vi "ScanAction.vi"(8 "error in (no error)":errorcluster caption="entrée d'erreur (pas d'erreur)", 9 "IndicePoint":i32, 10 "Dir":bool, 11 "Tools In":refnum<class "HeFlowMeter.lvclass"> caption="DNL_LabVIEW Object in") -> (0 "error out":errorcluster caption="sortie d'erreur", 2 "ScanParsOut":dbl[](array[numeric]), 3 "Tools Out":refnum<class "HeFlowMeter.lvclass"> caption="DNL_LabVIEW Object out")   [LabVIEW 2019, in "HeFlowMeter.lvclass"]
uses:
  HeFlowMeter.lvclass
  HeFlowMeter.lvclass/HeFlowMeter.ctl
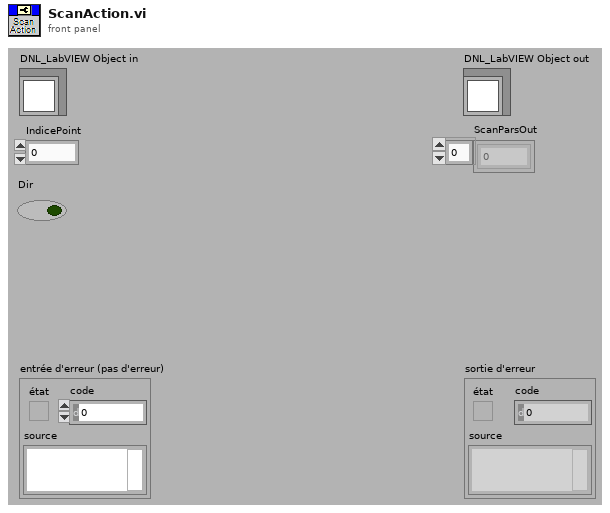
[diagram p1: front panel]
types:
  T1 = typedef "HeFlowMeter.lvclass/HeFlowMeter_Func.ctl" = enum16{"ReadFlow (m3h-1)"}
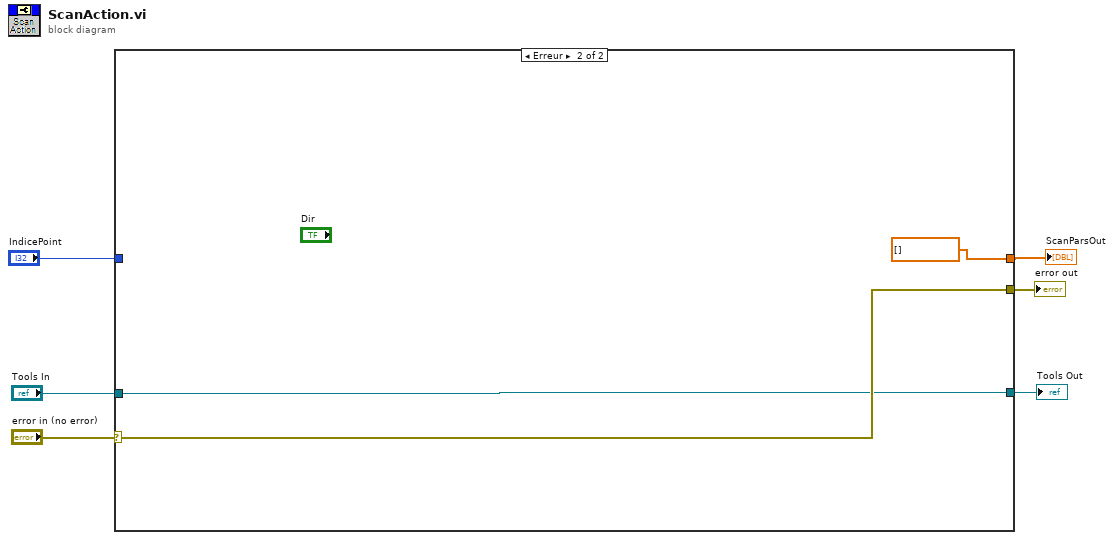
[diagram p0: block diagram]
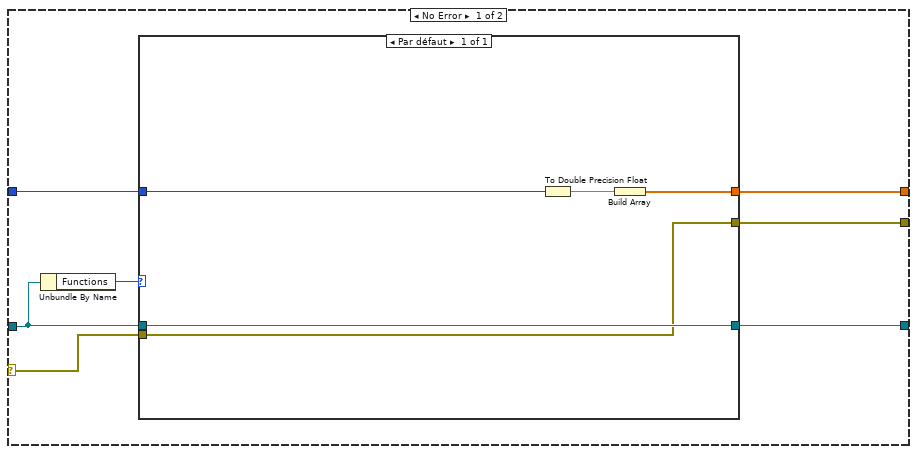
[diagram p2: hidden frame]
diagram:
  n1 = case shown="Erreur" "error in (no error)" {
    selector: "error in (no error)" -> [w10 w21]
    tunnel: "Tools In" -> [w11 w20]
    tunnel: [w9 dbl[] []] -> w1
    tunnel: [w8 w21] -> w4
    tunnel: [w7 w20] -> w3
    tunnel: "IndicePoint" -> [w12 _]
    frame No Error {
      n2 = Unbundle By Name(w11) -> ("Functions"=w13:T1)
      n3 = case shown="Par défaut" w13 {
        tunnel: [w14] -> w9
        tunnel: w12 -> [w18]
        tunnel: [w16] -> w7
        tunnel: w11 -> [w16]
        tunnel: w10 -> [w15]
        tunnel: [w15] -> w8
        frame Par défaut {
          n4 = To Double Precision Float(number=w18) -> (double precision float=w17:dbl)
          n5 = Build Array(w17) -> (w14:dbl[])
        }
      }
    }
    frame Error {
    }
  }
  "error out" <- w4
  "Tools Out" <- w3
  "ScanParsOut" <- w1
